vi "Read VRef.vi"(8 "error in (no error)":errorcluster, 11 "LINX-DAC8552 in":refnum<class "LINX-DAC8552.lvclass">) -> (0 "error out":errorcluster, 2 "VRef":dbl=5.0, 3 "LINX-DAC8552 out":refnum<class "LINX-DAC8552.lvclass">)   [LabVIEW 2020, in "LINX-DAC8552.lvclass"]
uses:
  LINX-DAC8552.lvclass
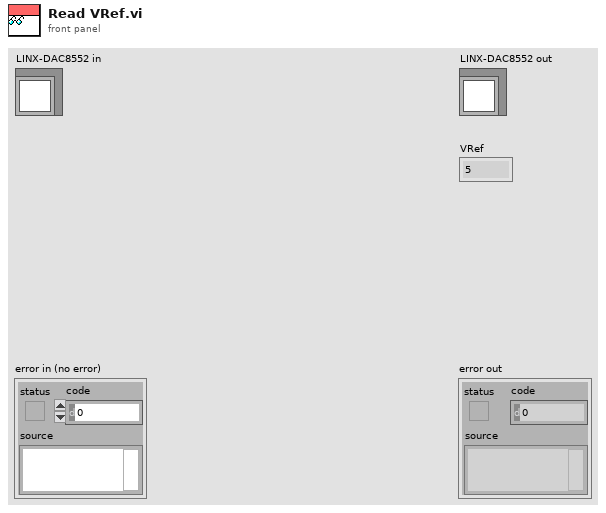
[diagram p1: front panel]
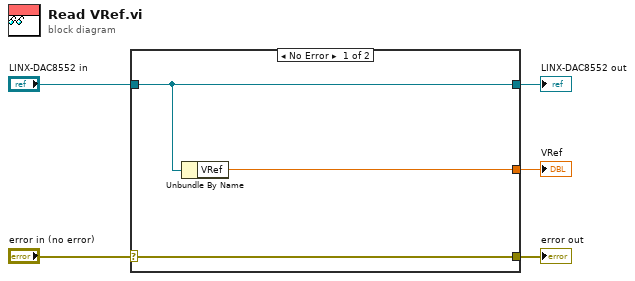
[diagram p0: block diagram]
diagram:
  n1 = case shown="No Error" "error in (no error)" {
    selector: "error in (no error)" -> [w8 w9]
    tunnel: [w8 w9] -> w4
    tunnel: [w7 w10] -> w2
    tunnel: "LINX-DAC8552 in" -> [w7 w10]
    tunnel: [w6 _] -> w1
    frame No Error {
      n2 = Unbundle By Name(w7) -> ("VRef"=w6:dbl)
    }
    frame Error {
    }
  }
  "error out" <- w4
  "LINX-DAC8552 out" <- w2
  "VRef" <- w1
